vi "Auto_Play_Grab.vi"() -> (1 "All Files":string[](array[string]), 2 "Auto Plays":string[](array[string]))   [LabVIEW 2020]
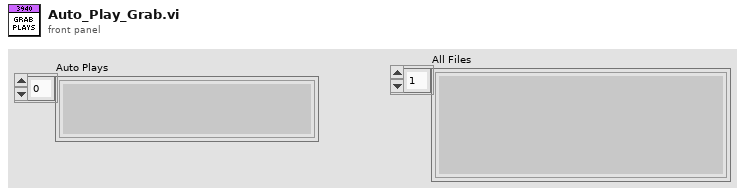
[diagram p1: front panel]
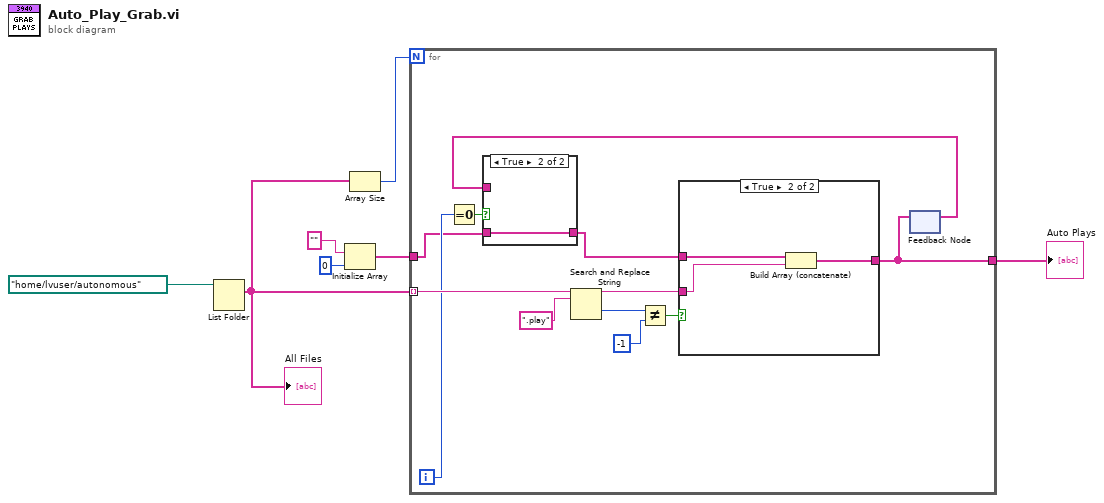
[diagram p0: block diagram]
diagram:
  n1 = List Folder(path=path "/home/lvuser/autonomous" ("file path (use dialog)")) -> (filenames=w5:string[])  [unwired: 3 in, 3 out]
  "All Files" <- w5
  n2 = Initialize Array("", 0 ("dimension size")) -> (w1:string[])
  n3 = Array Size(array=w5) -> (size(s)=w6:i32)
  n4 = for {
    N: w6 -> [_]
    tunnel: w5 -> [w19] mode=indexing
    tunnel: [w8] -> w2
    tunnel: w1 -> [w11]
    i -> [w12]
    n5 = Equal To 0?(x=w12) -> (x = 0?=w13:bool)
    n6 = Search and Replace String(input string=w19, search string=".play") -> (result string=w14:string, offset past replacement=w15:i32)  [unwired: 6 in, 2 out]
    n7 = Not Equal?(x=w15, y=-1) -> (x != y?=w17:bool)
    n8 = feedback #1() -> (w9:string[])  [unwired: 1 in]
    n9 = case shown="True" w13 {
      tunnel: w11 -> [_ w21]
      tunnel: [w20 w21] -> w10
      tunnel: w9 -> [w20 _]
      frame False {
      }
      frame True {
      }
    }
    n10 = case shown="True" w17 {
      tunnel: w14 -> [_ w25]
      tunnel: [w22 w24] -> w8
      tunnel: w10 -> [w22 w23]
      frame False {
      }
      frame True {
        n11 = Build Array (concatenate)(w23, w25) -> (w24:string[])
      }
    }
    n12 = feedback-in #1(w8) -> ()
  }
  "Auto Plays" <- w2
